vi "epl-neopixel-controller.vi"() -> ()   [LabVIEW 2020]
uses:
  epl-vi-lib/Utility VIs/Controls/KColorSliders/KColorSliders.xctl
  Typedefs/Neopixel-Parameters.ctl
  <vilib>/Instr/_visa.llb/VISA Find Search Mode.ctl
  <vilib>/Instr/_visa.llb/VISA Configure Serial Port (Instr).vi
panel:
  in  "Color":u32(xcontrol)
  in  "Toggle":bool
  out "status":bool
  in  "Port":u16(ring) items=["COM1", "CNCA0", "CNCB0"]
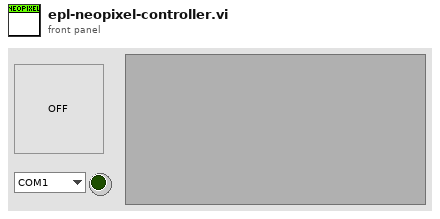
[diagram p1: front panel]
types:
  T1 = typedef "Neopixel-Parameters.ctl" = cluster{"COM port":string, "Color":u32}
  T2 = typedef "VISA Find Search Mode.ctl" = u32
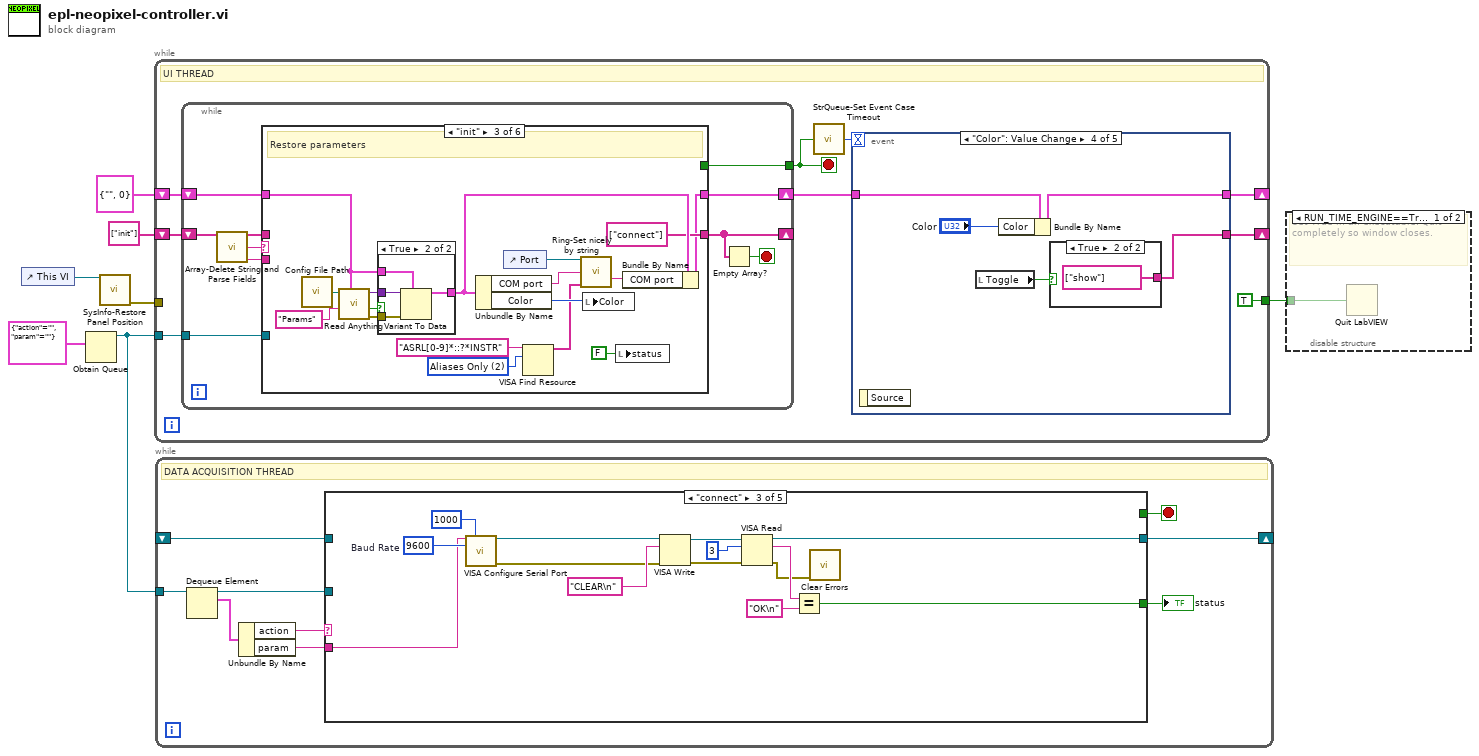
[diagram p0: block diagram]
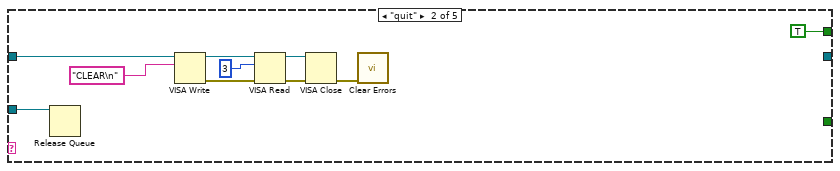
[diagram p3: hidden frame]
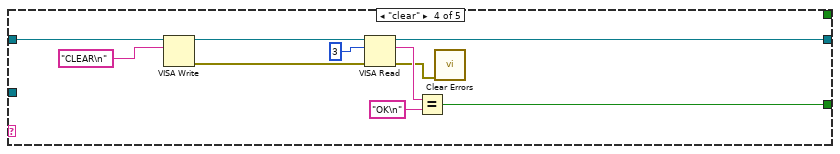
[diagram p4: hidden frame]
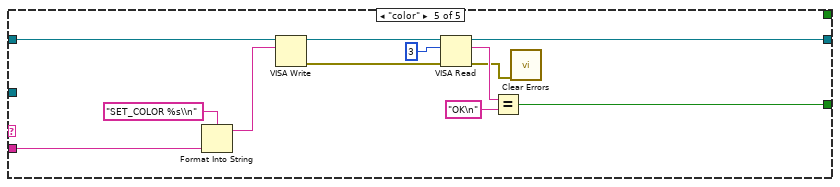
[diagram p5: hidden frame]
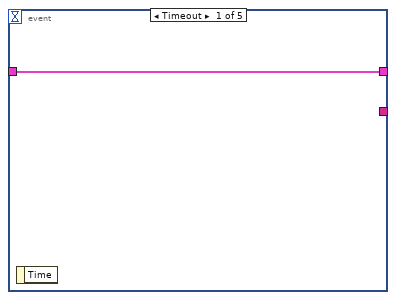
[diagram p6: hidden frame]
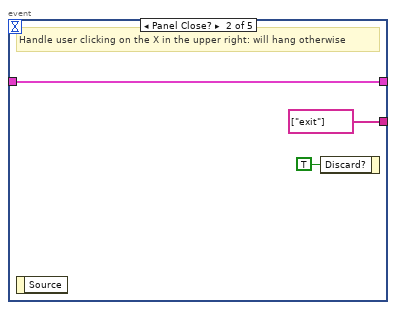
[diagram p7: hidden frame]
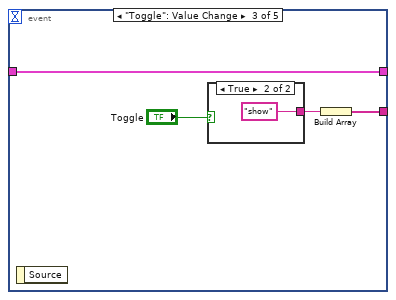
[diagram p8: hidden frame]
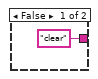
[diagram p9: hidden frame]
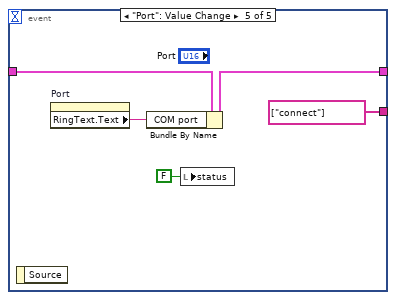
[diagram p11: hidden frame]
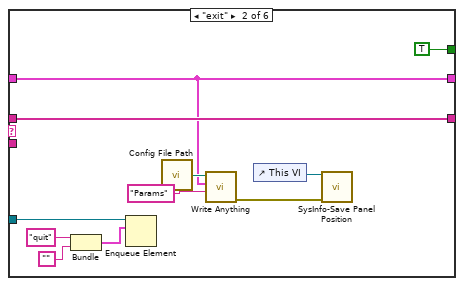
[diagram p13: hidden frame]
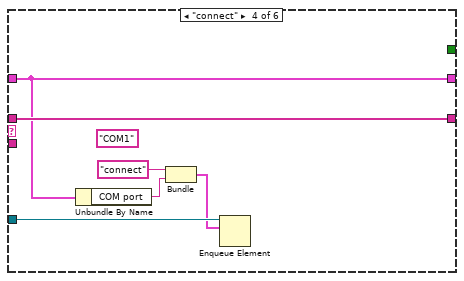
[diagram p15: hidden frame]
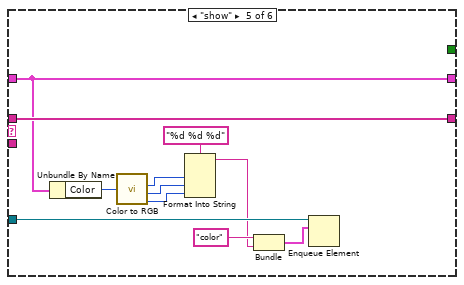
[diagram p16: hidden frame]
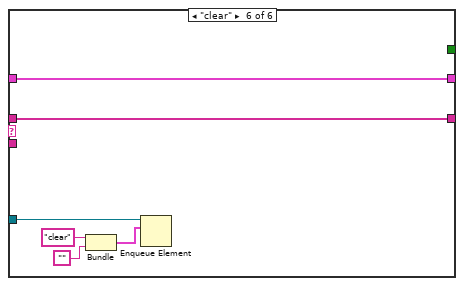
[diagram p17: hidden frame]
diagram:
  n1 = control-ref of="This VI"() -> (w2:refnum<vi>)
  n2 = Obtain Queue(element data type=cluster{"action":string, "param":string} {"action"="", "param"=""}) -> (queue out=w4:refnum<queue>)  [unwired: 4 in, 2 out]
  n3 = call "SysInfo-Restore Panel Position.vi"("VI Refnum"=w2) -> ("error out"=w1:errorcluster)  [unwired: 12 in, 2 out]
  n4 = while {
    shift-right: [w13] -> _
    shift-left: string[] ["init"] -> [w14]
    shift-right: [w10] -> _
    shift-left: T1 {"COM port"="", "Color"=0} ("\"Settings\" or \"Parameters\"") -> [w12]
    tunnel: [TRUE] -> w5
    tunnel: w4 -> [w8]
    tunnel: w1 -> [_]
    stop <- w16 stop-if-true
    # "UI THREAD"
    n5 = while {
      shift-right: [w47] -> _
      shift-left: w14 -> [w44]
      tunnel: [w45] -> w16
      shift-right: [w40] -> w11
      shift-left: w12 -> [w41]
      tunnel: w8 -> [w39]
      stop <- w46 stop-if-true
      n6 = call "Array-Delete String and Parse Fields.vi"("Array in"=w44) -> ("Array out"=w43:string[], "Field 1"=w42:string, "Field 2"=w38:string)  [unwired: 10 in, 2 out]
      n7 = case shown="\"init\"" w42 {
        tunnel: w43 -> [w49 w60 _ w88 w99 w105]
        tunnel: [w49 w60 string[] ["connect"] ("Array out") w88 w99 w105] -> w47
        tunnel: [_ TRUE _ _ _ _] -> w45
        tunnel: w41 -> [w48 w52 w74 w85 w95 w102]
        tunnel: [w48 w52 w66 w85 w95 w102] -> w40
        tunnel: w39 -> [_ w54 _ w86 w97 w103]
        tunnel: w38 -> [_ _ _ _ _ _]
        frame "", Default {
        }
        frame "exit" {
          n8 = Bundle("quit", "") -> (w50:cluster{string, string})  [unwired: 1 in]
          n9 = Enqueue Element(queue=w54, element=w50) -> ()  [unwired: 2 in, 3 out]
          n10 = call "Config File Path.vi"() -> ("Default config file name"=w56:path)  [unwired: 1 in]
          n11 = call "Write Anything.vi"("Section Name (Name of \"Anything\")"="Params" ("Section Name (Name of \"Anything\")"), "Anything"=w52, "Path (dialog)"=w56) -> ("Error Out"=w57:errorcluster)  [unwired: 7 in, 1 out]
          n12 = control-ref of="This VI"() -> (w58:refnum<vi>)
          n13 = call "SysInfo-Save Panel Position.vi"("VI Refnum"=w58, "error in (no error)"=w57) -> ()  [unwired: 13 in, 1 out]
        }
        frame "init" {
          w64 = T2 2 items=["Canonical Names Only"=0, "Aliases Only"=2, "Include Matching Aliases"=3, "Include All Aliases"=4] ("Search Mode")
          # "Restore parameters"
          n14 = call "Config File Path.vi"() -> ("Default config file name"=w77:path)  [unwired: 1 in]
          n15 = call "Read Anything.vi"("Type of Anything"=w74, "Section Name (Name of \"Type of Anything\")"="Params" ("Section Name (Name of \"Type of Anything\")"), "Path (dialog)"=w77) -> ("Error Out"=w72:errorcluster, "Found?"=w73:bool, "Anything"=w75:variant)  [unwired: 6 in]
          n16 = case shown="True" w73 {
            tunnel: w75 -> [_ w81]
            tunnel: w74 -> [w78 w80]
            tunnel: w72 -> [_ w82]
            tunnel: [w78 w79] -> w71
            frame False {
            }
            frame True {
              n17 = Variant To Data(error in=w82, type=w80, Variant=w81) -> (data=w79:T1)  [unwired: 1 out]
            }
          }
          n18 = Unbundle By Name(w71) -> ("COM port"=w68:string, "Color"=w70:u32)
          n19 = control-ref of="Port"() -> (w67:refnum<vi>)
          n20 = VISA Find Resource(10:w64, 11:"ASRL[0-9]*::?*INSTR" ("expression (\"?*\")")) -> (3:w62:string[])  [unwired: 1 in, 2 out]
          n21 = call "Ring-Set nicely by string.vi"("Ring in"=w67, "Device"=w68, "Strings []"=w62) -> ("Selection"=w65:string)  [unwired: 8 in, 4 out]
          n22 = local write "Color"(w70) -> ()
          n23 = local write "status"(FALSE ("status")) -> ()
          n24 = Bundle By Name(cluster=w71, "COM port"=w65) -> (w66:T1)
        }
        frame "connect" {
          (unwired) "COM1"
          n25 = Unbundle By Name(w85) -> ("COM port"=w83:string)
          n26 = Bundle("connect", "COM port"=w83) -> (w84:cluster{string, "COM port":string})  [unwired: 1 in]
          n27 = Enqueue Element(queue=w86, element=w84) -> ()  [unwired: 2 in, 3 out]
        }
        frame "show" {
          n28 = Unbundle By Name(w95) -> ("Color"=w90:u32)
          n29 = call <vilib>:"Color to RGB.vi"("Color"=w90) -> ("R"=w93:u8, "G"=w92:u8, "B"=w91:u8)  [unwired: 1 out]
          n30 = Format Into String(format string="%d %d %d", w93, w92, w91) -> (resulting string=w89:string)  [unwired: 2 in, 1 out]
          n31 = Bundle("color", w89) -> (w96:cluster{string, string})  [unwired: 1 in]
          n32 = Enqueue Element(queue=w97, element=w96) -> ()  [unwired: 2 in, 3 out]
        }
        frame "clear" {
          n33 = Bundle("clear", "") -> (w100:cluster{string, string})  [unwired: 1 in]
          n34 = Enqueue Element(queue=w103, element=w100) -> ()  [unwired: 2 in, 3 out]
        }
      }
      n35 = Empty Array?(array=w47) -> (empty?=w46:bool)
    }
    n36 = call "StrQueue-Set Event Case Timeout.vi"("Quit"=w16) -> ("timeout"=w15:i32)  [unwired: 14 in]
    n37 = event shown="[3] \"Color\": Value Change" {
      selector: _ -> [_ _ _ _ _]
      dyn-events: _ -> [_ _ _ _ _]
      timeout: w15 -> [_ _ _ _ _]
      tunnel: [_ string[] ["exit"] w22 w29 string[] ["connect"]] -> w13
      tunnel: w11 -> [w17 w18 w24 w31 w37]
      tunnel: [w17 w18 w24 w30 w36] -> w10
      event Timeout {
        n38 = event-data() -> ()  [unwired: 1 in, 1 out]
      }
      event Panel Close? {
        # "Handle user clicking on the X in the upper right: will hang otherwise"
        n39 = event-data() -> ()  [unwired: 1 in, 1 out]
        n40 = event-data("Discard?"=TRUE) -> ()  [unwired: 1 in, 1 out]
      }
      event "Toggle": Value Change {
        n41 = event-data() -> ()  [unwired: 1 in, 1 out]
        n42 = case shown="True" "Toggle" {
          tunnel: ["clear" "show"] -> w23
          frame False {
          }
          frame True {
          }
        }
        n43 = Build Array(w23) -> (w22:string[])
      }
      event "Color": Value Change {
        n44 = event-data() -> ()  [unwired: 1 in, 1 out]
        n45 = local read "Toggle"() -> (w28:bool)
        n46 = Bundle By Name(cluster=w31, "Color"="Color") -> (w30:T1)
        n47 = case shown="True" w28 {
          tunnel: [_ string[] ["show"]] -> w29
          frame False {
          }
          frame True {
          }
        }
      }
      event "Port": Value Change {
        n48 = event-data() -> ()  [unwired: 1 in, 1 out]
        n49 = property on="Port" class="Ring (strict)"() -> ("RingText.Text"=w34:string)  [unwired: 2 in, 2 out]
        n50 = Bundle By Name(cluster=w37, "COM port"=w34) -> (w36:T1)
        n51 = local write "status"(FALSE ("status")) -> ()
      }
    }
  }
  n52 = while {
    tunnel: w4 -> [w114]
    shift-right: [w108] -> _
    shift-left: _ -> [w107]
    stop <- w111 stop-if-true
    # "DATA ACQUISITION THREAD"
    n53 = Dequeue Element(queue=w114) -> (queue out=w109:refnum<queue>, element=w110:cluster{"action":string, "param":string})  [unwired: 2 in, 2 out]
    n54 = Unbundle By Name(w110) -> ("action"=w113:string, "param"=w112:string)
    n55 = case shown="\"connect\"" w113 {
      tunnel: w112 -> [_ _ w138 _ w158]
      tunnel: [_ TRUE _ _ _] -> w111
      tunnel: w109 -> [_ w124 _ _ _]
      tunnel: [w115 _ w136 w142 w153] -> w108
      tunnel: w107 -> [w115 w122 _ w148 w161]
      tunnel: [_ _ w126 w140 w150] -> w106
      frame "", Default {
      }
      frame "quit" {
        n56 = Release Queue(queue=w124) -> ()  [unwired: 2 in, 3 out]
        n57 = VISA Write(VISA resource name=w122, write buffer="CLEAR\n" ("format string")) -> (VISA resource name out=w119:refnum<visa-resource-name>, error out=w117:errorcluster)  [unwired: 1 in, 1 out]
        n58 = VISA Read(VISA resource name=w119, byte count=u32 3, error in (no error)=w117) -> (VISA resource name out=w118:refnum<visa-resource-name>, error out=w116:errorcluster)  [unwired: 2 out]
        n59 = VISA Close(VISA resource name=w118, error in (no error)=w116) -> (error out=w121:errorcluster)
        n60 = call <vilib>:"Clear Errors.vi"("error in (no error)"=w121) -> ()  [unwired: 5 in, 2 out]
      }
      frame "connect" {
        w139 = u32 9600  # Baud Rate
        n61 = call-poly "VISA Configure Serial Port"("VISA resource name"=w138, "timeout (10sec)"=u32 1000, "baud rate (9600)"=w139) -> ("VISA resource name out"=w135:refnum<visa-resource-name>, "error out"=w127:errorcluster)  [unwired: 6 in, 5 out]
        n62 = VISA Write(VISA resource name=w135, write buffer="CLEAR\n" ("format string"), error in (no error)=w127) -> (VISA resource name out=w130:refnum<visa-resource-name>, error out=w129:errorcluster)  [unwired: 1 out]
        n63 = VISA Read(VISA resource name=w130, byte count=u32 3, error in (no error)=w129) -> (VISA resource name out=w136:refnum<visa-resource-name>, read buffer=w132:string, error out=w128:errorcluster)  [unwired: 1 out]
        n64 = Equal?(x=w132, y="OK\n") -> (x = y?=w126:bool)
        n65 = call <vilib>:"Clear Errors.vi"("error in (no error)"=w128) -> ()  [unwired: 5 in, 2 out]
      }
      frame "clear" {
        n66 = VISA Write(VISA resource name=w148, write buffer="CLEAR\n" ("format string")) -> (VISA resource name out=w143:refnum<visa-resource-name>, error out=w141:errorcluster)  [unwired: 1 in, 1 out]
        n67 = VISA Read(VISA resource name=w143, byte count=u32 3, error in (no error)=w141) -> (VISA resource name out=w142:refnum<visa-resource-name>, read buffer=w146:string, error out=w144:errorcluster)  [unwired: 1 out]
        n68 = Equal?(x=w146, y="OK\n") -> (x = y?=w140:bool)
        n69 = call <vilib>:"Clear Errors.vi"("error in (no error)"=w144) -> ()  [unwired: 5 in, 2 out]
      }
      frame "color" {
        n70 = Format Into String(format string="SET_COLOR %s\\n", w158) -> (resulting string=w159:string)  [unwired: 2 in, 1 out]
        n71 = VISA Write(VISA resource name=w161, write buffer=w159) -> (VISA resource name out=w154:refnum<visa-resource-name>, error out=w152:errorcluster)  [unwired: 1 in, 1 out]
        n72 = VISA Read(VISA resource name=w154, byte count=u32 3, error in (no error)=w152) -> (VISA resource name out=w153:refnum<visa-resource-name>, read buffer=w156:string, error out=w151:errorcluster)  [unwired: 1 out]
        n73 = Equal?(x=w156, y="OK\n") -> (x = y?=w150:bool)
        n74 = call <vilib>:"Clear Errors.vi"("error in (no error)"=w151) -> ()  [unwired: 5 in, 2 out]
      }
    }
    "status" <- w106
  }
  n75 = disable-structure shown="RUN_TIME_ENGINE==True" {
    disable-tunnel: w5 -> [w162 _]
    frame condition #0 {
      # "Set True in an executable. Quit completely so window closes."
      n76 = Quit LabVIEW(quit? (T)=w162) -> ()
    }
    frame condition #1 (active) {
      # "Running in LabVIEW development system. Leaves window open"
    }
  }
